vi "Do.vi"(8 "error in (no error)":errorcluster, 10 "Numeric":dbl, 11 "Object In":refnum<class "Sub.lvclass">) -> (0 "error out":errorcluster, 2 "String":string, 3 "Object Out":refnum<class "Sub.lvclass">)   [LabVIEW 2014, in "Sub.lvclass"]
uses:
  Sub.lvclass
  Sub.lvclass/Sub.ctl
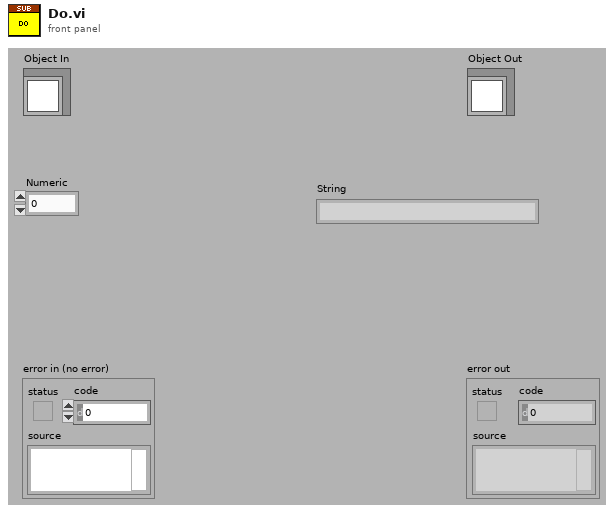
[diagram p1: front panel]
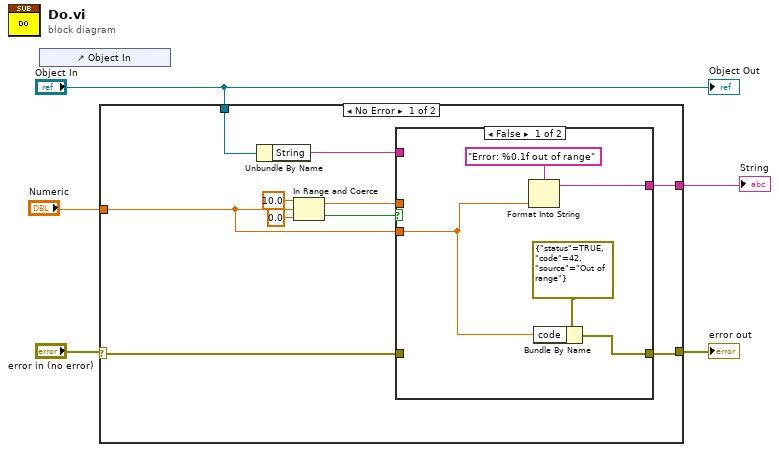
[diagram p0: block diagram]
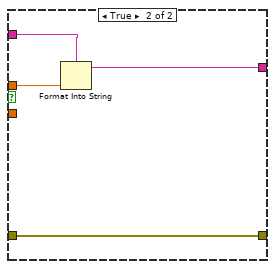
[diagram p2: hidden frame]
diagram:
  n1 = control-ref of="Object In"() -> ()  [unwired: 1 out]
  n2 = case shown="No Error" "error in (no error)" {
    selector: "error in (no error)" -> [w11 w25]
    tunnel: [w10 w25] -> w4
    tunnel: "Numeric" -> [w8 _]
    tunnel: [w12 _] -> w2
    tunnel: "Object In" -> [w7 _]
    frame No Error {
      n3 = Unbundle By Name(w7) -> ("String"=w9:string)
      n4 = In Range and Coerce(upper limit=10.0, x=w8, lower limit=0.0) -> (coerced(x)=w13:dbl, In Range?=w6:bool)
      n5 = case shown="False" w6 {
        tunnel: w13 -> [_ w24]
        tunnel: [w19 w23] -> w12
        tunnel: w11 -> [_ w22]
        tunnel: [w16 w22] -> w10
        tunnel: w9 -> [_ w21]
        tunnel: w8 -> [w18 _]
        frame False {
          n6 = Format Into String(format string="Error: %0.1f out of range", w18) -> (resulting string=w19:string)  [unwired: 2 in, 1 out]
          n7 = Bundle By Name(cluster=errorcluster {"status"=TRUE, "code"=42, "source"="Out of range"} ("error IO"), "code"=w18) -> (w16:errorcluster)
        }
        frame True {
          n8 = Format Into String(format string=w21, w24) -> (resulting string=w23:string)  [unwired: 2 in, 1 out]
        }
      }
    }
    frame Error {
    }
  }
  "error out" <- w4
  "String" <- w2
  "Object Out" <- "Object In"
